vi "Z Aux Direct Move Op Multi.vi"(7 "ivalue":i32, 8 "error in (no error)":errorcluster caption="错误输入（无错误）", 9 "ioutnumend":i32, 10 "ioutnumfirst":i32, 11 "handle":u32) -> (0 "error out":errorcluster caption="错误输出", 2 "function return":i32, 3 "handle out":u32)   [LabVIEW 2015, in "zauxdll.lvlib"]
doc: "int32 __stdcall ZAux_Direct_MoveOpMulti(ZMC_HANDLE handle, int ioutnumfirst, int ioutnumend, int ivalue);"
uses:
  zauxdll.lvlib
  zauxdll.dll
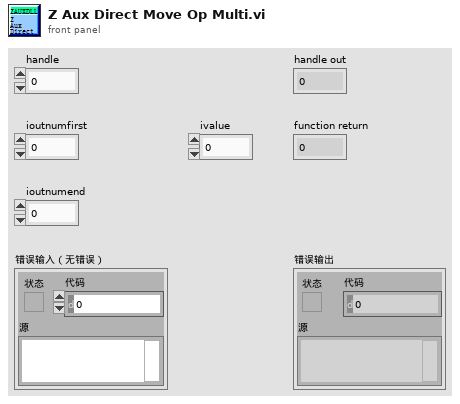
[diagram p1: front panel]
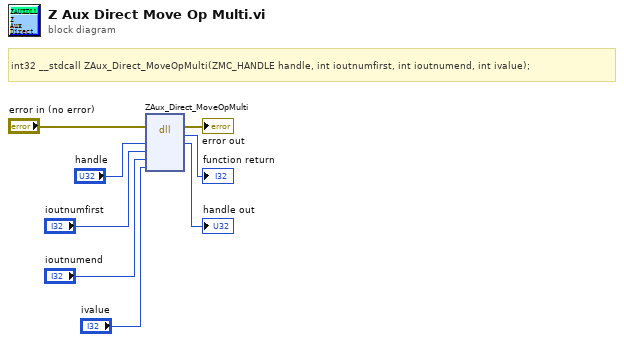
[diagram p0: block diagram]
diagram:
  # "int32 __stdcall ZAux_Direct_MoveOpMulti(ZMC_HANDLE handle, int ioutnumfirst, int ioutnumend, int ivalue);"
  n1 = dll-call lib="C:/Users/VIC/Desktop/GOGORO_Oringnal - Panasonic/system/LLB/zmotion/zaux/zauxdll.*" fn="ZAux_Direct_MoveOpMulti"(error in="error in (no error)", "handle"="handle", "ioutnumfirst"="ioutnumfirst", "ioutnumend"="ioutnumend", "ivalue"="ivalue") -> (error out=→"error out":errorcluster, →"function return":i32, "handle"=→"handle out":u32)  [unwired: 5 in, 1 out]
